vi "Do.vi"(8 "error in":errorcluster, 10 "Actor in":refnum<class "Actor.lvclass">, 11 "Change Filter Position MSG":refnum<class "Change Filter Position MSG.lvclass">) -> (0 "error out":errorcluster, 2 "Actor out":refnum<class "Actor.lvclass">)   [LabVIEW 2016, in "Controller.lvlib" / "Change Filter Position MSG.lvclass"]
doc: "(<B>Filename</B>: Actor Framework.lvlib:Message.lvclass:Do.vi)\n\nDefines what a message does when it is received by an actor. Generally, a message instructs an actor to invoke one of its methods. By default, this method does nothing. A child class must override it to define behavior. Create a child class by using the Actor Framework Message Maker dialog box."
uses:
  Change Filter Position MSG.lvclass
  <vilib>/ActorFramework/Actor/Actor.lvclass
  Change Filter Position MSG.lvclass/Change Filter Position MSG.ctl
  gController.lvclass
  C:/Program Files (x86)/National Instruments/LabVIEW 2016/vi.lib/ActorFramework/Actor/Actor.lvclass
  Forward Command/Forward Command MSG.lvclass
  C:/Program Files (x86)/National Instruments/LabVIEW 2016/vi.lib/ActorFramework/Message/Message.lvclass
  <vilib>/MSR Consulting, LLC/General Reuse/PAS/Commands/Change Filter State CMD/Change Filter State CMD.lvclass
  C:/Program Files (x86)/National Instruments/LabVIEW 2016/vi.lib/MSR Consulting, LLC/General Reuse/Command/Command.lvclass
  <vilib>/MSR Consulting, LLC/General Reuse/CRDS/Commands/Change Filter State CMD/Change Filter State CMD.lvclass
  Global FPGA DO.ctl
  <vilib>/MSR Consulting, LLC/General Reuse/CRDS/Commands/Change Filter State CMD/Change Filter State CMD.lvclass/Change Filter State CMD.ctl
  <vilib>/MSR Consulting, LLC/General Reuse/PAS/Commands/Change Filter State CMD/Change Filter State CMD.lvclass/Change Filter State CMD.ctl
  Forward Command/Forward Command MSG.lvclass/Forward Command MSG.ctl
  <vilib>/ActorFramework/Message Enqueuer/Message Enqueuer.lvclass/Message Enqueuer.ctl
  gController.lvclass/gController.ctl
  Session/Raw FPGA/FPGA Session.lvclass/FPGA Session.ctl
  Read FPGA Session.vi
  Session/Raw FPGA/Read FPGA Ref.vi
  Forward Command/Write CMD.vi
  Forward Command/Write id.vi
  <vilib>/MSR Consulting, LLC/General Reuse/PAS/Commands/Change Filter State CMD/Write cell.vi
  <vilib>/MSR Consulting, LLC/General Reuse/PAS/Commands/Change Filter State CMD/Write state.vi
  <vilib>/MSR Consulting, LLC/General Reuse/CRDS/Commands/Change Filter State CMD/Write cell.vi
  <vilib>/MSR Consulting, LLC/General Reuse/CRDS/Commands/Change Filter State CMD/Write state.vi
  Global DO.vi
  <vilib>/rvi/errors/niLvFpgaAdjustHostInterfaceError.vi
  <vilib>/Utility/error.llb/Error Cluster From Error Code.vi
  <vilib>/ActorFramework/Message Priority Queue/Priority Enqueue.vi
  FPGA Ref.ctl
  <vilib>/rvi/interface/nirviReadWriteControl/nirviReadWriteControl.xnode
  FPGA Bitfiles/server_v0_2_1_3.lvbitx
  Session/Raw FPGA/FPGA Session.lvclass
  <vilib>/ActorFramework/Message Enqueuer/Message Enqueuer.lvclass
  NiFpgaLv.dll
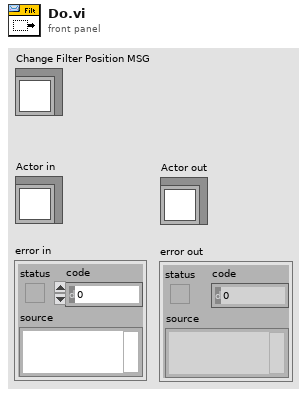
[diagram p1: front panel]
types:
  T1 = typedef "Global FPGA DO.ctl" = enum16{"pas_laser_relay_1", "pas_heater_1", "pas_heater_2", "pas_laser_relay_2", "pas_spk_enable_1", "pas_spk_enable_2", "hanbay_pos", "fan_enable", "crd_laser_enable", "crd_heater_enable", "vacuum_pump", "ac_spare", "uv_enable", "solenoid_1", "solenoid_2", "spare_dc_relay_1", "usb_hub_relay", "spare_dc_relay_2", "fp_aux_1", "fp_aux_2"}
  T2 = typedef "FPGA Ref.ctl" = refnum<k20>
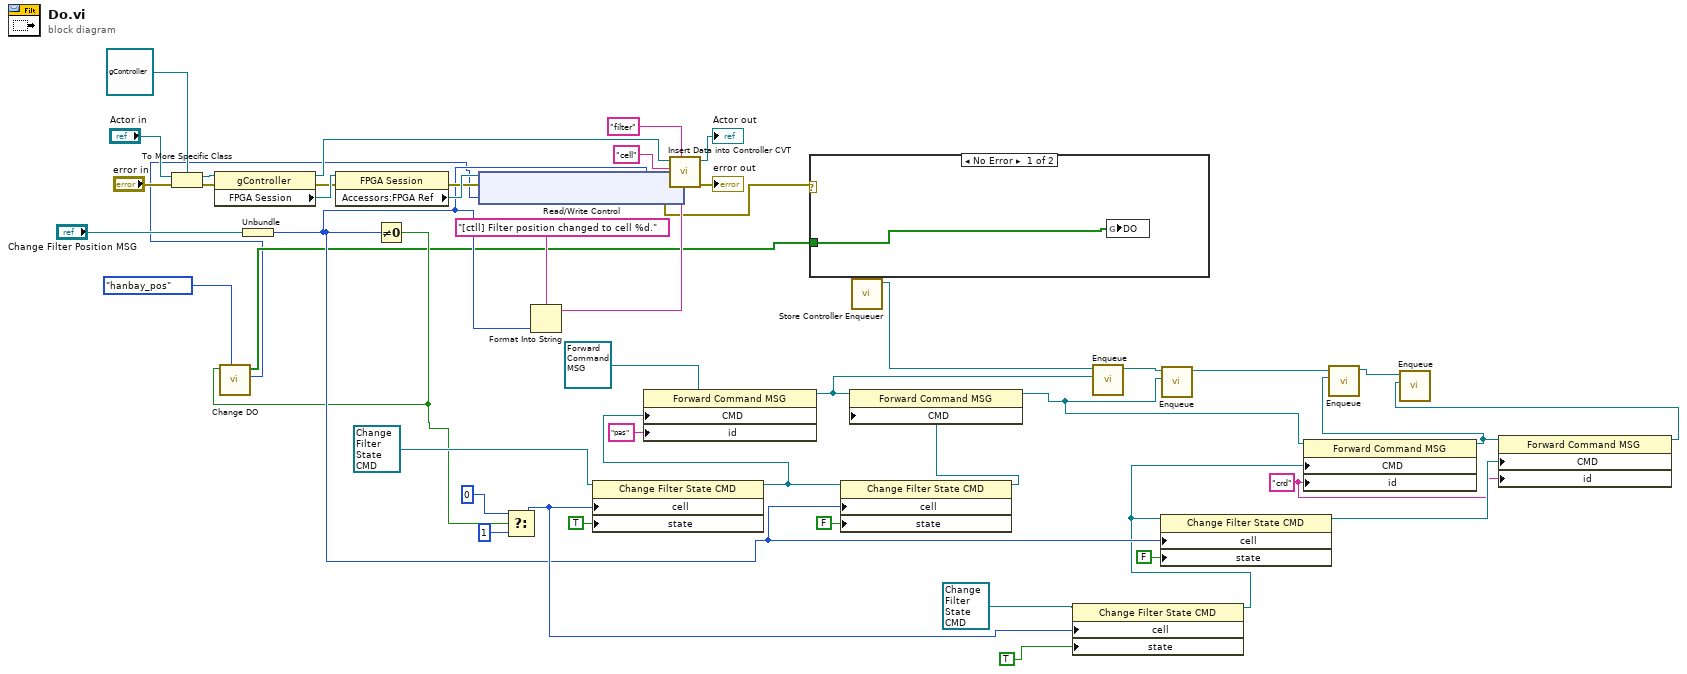
[diagram p0: block diagram]
diagram:
  w10 = "crd" ("id")
  n1 = To More Specific Class(target class=refnum<class "gController.lvclass"> refnum ("Controller.lvlib:gController"), reference="Actor in", error in="error in") -> (specific class reference=w44:refnum<class "gController.lvclass">, error out=w36:errorcluster)
  n2 = property class="gController"(reference=w44, error in=w36) -> (reference out=w43:refnum<class "gController.lvclass">, error out=w32:errorcluster, "FPGA Session"=w35:refnum<data-value>)
  n3 = Unbundle("Change Filter Position MSG") -> (w15:u8)
  n4 = property class="FPGA Session"(reference=w35, error in=w32) -> (error out=w33:errorcluster, "Accessors:FPGA Ref"=w34:T2)  [unwired: 1 out]
  n5 = Not Equal To 0?(x=w15) -> (x != 0?=w3:bool)
  n6 = call "Change DO.vi"("DO"=Global_FPGA_DO."hanbay_pos", "val_in"=w3) -> ("DO Long Out"=w1:u32, "DO Out"=w2:bool[])  [unwired: 8 in]
  n7 = xnode "Read/Write Control"("FPGA VI Reference In"=w34, "error in"=w33, "DO"=w1) -> ("error out"=w5:errorcluster)  [unwired: 1 out]
  n8 = Select(t=u8 0 ("Cell"), s=w3, f=u8 1) -> (s? t:f=w17:u8)
  n9 = Format Into String(format string="[ctll] Filter position changed to cell %d.", w15) -> (resulting string=w38:string)  [unwired: 2 in, 1 out]
  n10 = property class="Change Filter State CMD"(reference=refnum<class "Change Filter State CMD.lvclass"> refnum ("PAS Library.lvlib:Change Filter State CMD"), "cell"=w17, "state"=TRUE) -> (reference out=w23:refnum<class "Change Filter State CMD.lvclass">)  [unwired: 1 in, 1 out]
  n11 = property class="Forward Command MSG"(reference=refnum<class "Forward Command MSG.lvclass"> refnum ("Controller.lvlib:Forward Command MSG"), "CMD"=w23, "id"="pas") -> (reference out=w21:refnum<class "Forward Command MSG.lvclass">)  [unwired: 1 in, 1 out]
  n12 = call "Insert Data into Controller CVT.vi"("Update MSG"=w38, "Group"="filter", "error in"=w5, "Data"=w15, "tag"="cell", "Actor in"=w43) -> ("error out"=→"error out":errorcluster, "Actor Out"=→"Actor out":refnum<class "Actor.lvclass">)  [unwired: 4 in]
  n13 = case shown="No Error" w5 {
    tunnel: w2 -> [w48 _]
    frame No Error {
      n14 = global write "Global DO.vi" "DO"(w48) -> ()
    }
    frame Error {
    }
  }
  n15 = property class="Change Filter State CMD"(reference=w23, "cell"=w15, "state"=FALSE) -> (reference out=w22:refnum<class "Change Filter State CMD.lvclass">)  [unwired: 1 in, 1 out]
  n16 = property class="Forward Command MSG"(reference=w21, "CMD"=w22) -> (reference out=w13:refnum<class "Forward Command MSG.lvclass">)  [unwired: 1 in, 1 out]
  n17 = call "Store Controller Enqueuer.vi"() -> ("Controller Enqueuer Out"=w20:refnum<class "Message Enqueuer.lvclass">)  [unwired: 11 in]
  n18 = property class="Change Filter State CMD"(reference=refnum<class "Change Filter State CMD.lvclass"> refnum ("CRDS Lib.lvlib:Change Filter State CMD"), "cell"=w17, "state"=TRUE) -> (reference out=w12:refnum<class "Change Filter State CMD.lvclass">)  [unwired: 1 in, 1 out]
  n19 = call <vilib>:"Enqueue.vi"("Message"=w21, "Message Enqueuer in"=w20) -> ("Message Enqueuer out"=w19:refnum<class "Message Enqueuer.lvclass">)  [unwired: 8 in, 1 out]
  n20 = property class="Change Filter State CMD"(reference=w12, "cell"=w15, "state"=FALSE) -> (reference out=w11:refnum<class "Change Filter State CMD.lvclass">)  [unwired: 1 in, 1 out]
  n21 = call <vilib>:"Enqueue.vi"("Message"=w13, "Message Enqueuer in"=w19) -> ("Message Enqueuer out"=w9:refnum<class "Message Enqueuer.lvclass">)  [unwired: 8 in, 1 out]
  n22 = property class="Forward Command MSG"(reference=w13, "CMD"=w12, "id"=w10) -> (reference out=w8:refnum<class "Forward Command MSG.lvclass">)  [unwired: 1 in, 1 out]
  n23 = call <vilib>:"Enqueue.vi"("Message"=w8, "Message Enqueuer in"=w9) -> ("Message Enqueuer out"=w7:refnum<class "Message Enqueuer.lvclass">)  [unwired: 8 in, 1 out]
  n24 = property class="Forward Command MSG"(reference=w8, "CMD"=w11, "id"=w10) -> (reference out=w6:refnum<class "Forward Command MSG.lvclass">)  [unwired: 1 in, 1 out]
  n25 = call <vilib>:"Enqueue.vi"("Message"=w6, "Message Enqueuer in"=w7) -> ()  [unwired: 8 in, 2 out]
